vi "选择产品.vi"   [LabVIEW 2019]
panel:
  # "请选择产品"
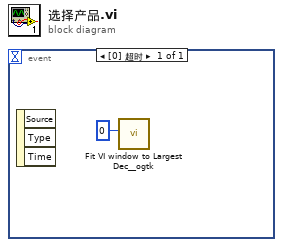
[diagram p0: block diagram]
diagram:
  n1 = event shown="[0] 超时" {
    selector: _ -> [_]
    dyn-events: _ -> [_]
    timeout: _ -> [_]
    event Timeout {
      n2 = event-data() -> ()  [unwired: 1 in, 3 out]
      n3 = call "Fit VI window to Largest Dec__ogtk.vi"("border spacing (2 px)"=0) -> ()  [unwired: 5 in, 2 out]
    }
  }
